vi "example_2_5_b.vi"() -> ()   [LabVIEW 2018]
panel:
  out "Digital Indicators Array":dbl[](array[numeric]) format="%.2f"
  in  "Knob":dbl(knob) scale=0.0..10.0 scale format="%.1f"
  in  "Digital Control":dbl format="%.2f"
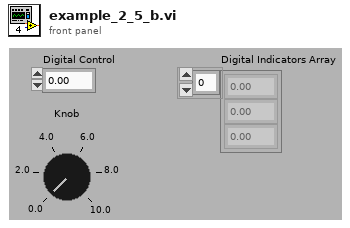
[diagram p1: front panel]
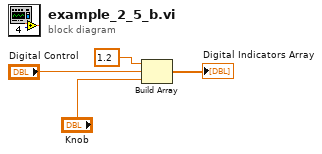
[diagram p0: block diagram]
diagram:
  n1 = Build Array(1.2 ("Input Element"), "Digital Control", "Knob") -> (→"Digital Indicators Array":dbl[])
